vi "EJEM11.vi"() -> ()   [LabVIEW 2013]
panel:
  out "text":string
  out "error out":errorcluster
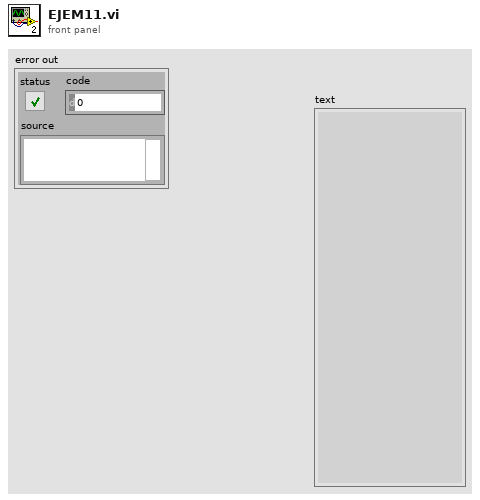
[diagram p1: front panel]
types:
  T1 = enum16{"open", "replace", "create", "open or create", "replace or create", "replace or create with confirmation"}
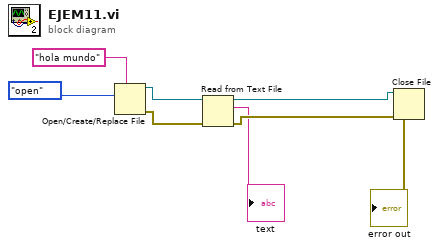
[diagram p0: block diagram]
diagram:
  n1 = Open/Create/Replace File(prompt="hola mundo", operation (0:open)=T1."open") -> (refnum out=w4:refnum<file>, error out=w7:errorcluster)  [unwired: 4 in, 1 out]
  n2 = Read from Text File(file (use dialog)=w4, error in=w7) -> (refnum out=w5:refnum<file>, text=→"text":string, error out=w6:errorcluster)  [unwired: 2 in, 1 out]
  n3 = Close File(refnum=w5, error in=w6) -> (error out=→"error out":errorcluster)  [unwired: 1 out]
